vi "Untitled 1.vi"() -> ()   [LabVIEW 2022 SP3]
panel:
  out "QUOITENT":dbl
  out "PRODUCT":dbl
  out "DIFFERENCE":dbl
  out "SUM":dbl
  in  "B":dbl
  in  "A":dbl
  # "CALCULATOR"
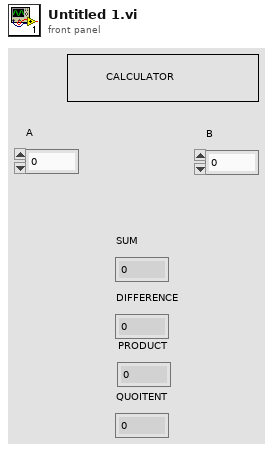
[diagram p1: front panel]
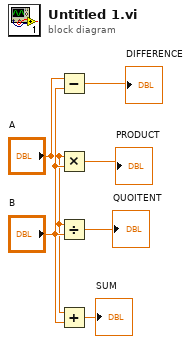
[diagram p0: block diagram]
diagram:
  n1 = Subtract(x="A", y="B") -> (x-y=→"DIFFERENCE":dbl)
  n2 = Multiply(x="A", y="B") -> (x*y=→"PRODUCT":dbl)
  n3 = Divide(x="A", y="B") -> (x/y=→"QUOITENT":dbl)
  n4 = Add(x="A", y="B") -> (x+y=→"SUM":dbl)
